vi "Updata LeafNumber.vi"(8 "error in (no error)":errorcluster caption="错误输入（无错误）", 11 "PanelLinkNode 输入":refnum<class "PanelLinkNode.lvclass"> caption="DNL_LabVIEW Object in") -> (0 "error out":errorcluster caption="错误输出", 2 "*Leafs":u8, 3 "PanelLinkNode 输出":refnum<class "PanelLinkNode.lvclass"> caption="DNL_LabVIEW Object out")   [LabVIEW 2013, in "PanelLinkNode.lvclass"]
uses:
  PanelLinkNode.lvclass
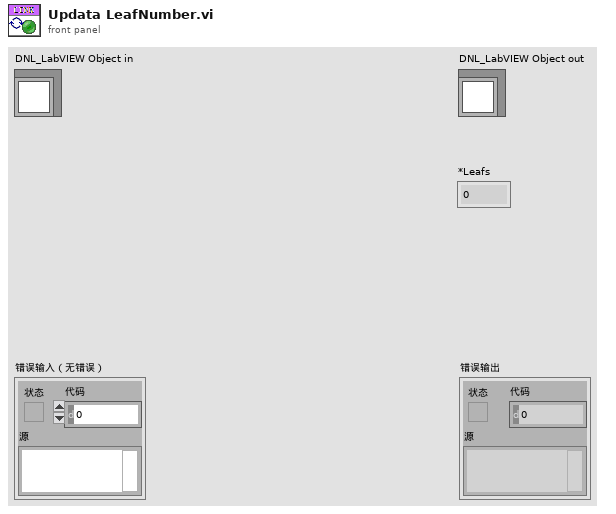
[diagram p1: front panel]
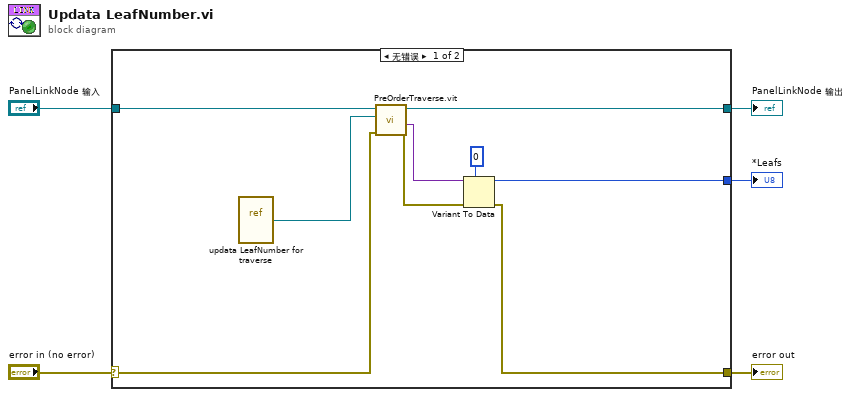
[diagram p0: block diagram]
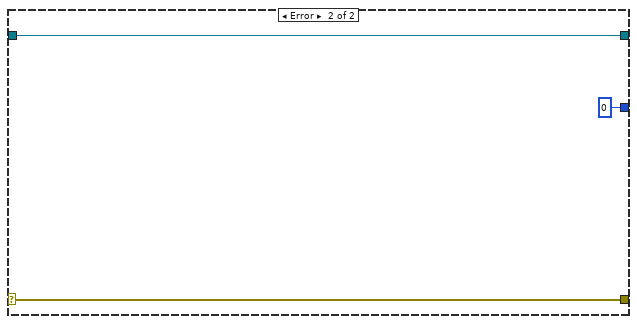
[diagram p2: hidden frame]
diagram:
  n1 = case shown="无错误" "error in (no error)" {
    selector: "error in (no error)" -> [w7 w17]
    tunnel: [w6 w17] -> w4
    tunnel: [w14 w16] -> w2
    tunnel: "PanelLinkNode 输入" -> [w9 w16]
    tunnel: [w11 u8 0] -> w1
    frame No Error {
      n2 = vi-ref "updata LeafNumber for traverse.vi"() -> (w10:refnum<vi>)
      n3 = call-dynamic "PreOrderTraverse.vit"("error in"=w7, "vi reference"=w10, "PanelLinkNode 输入"=w9) -> ("error out"=w8:errorcluster, "Data out"=w13:variant, "PanelLinkNode 输出"=w14:refnum<class "PanelLinkNode.lvclass">)  [unwired: 5 in, 1 out]
      n4 = Variant To Data(error in=w8, type=u8 0, Variant=w13) -> (data=w11:u8, error out=w6:errorcluster)
    }
    frame Error {
    }
  }
  "error out" <- w4
  "PanelLinkNode 输出" <- w2
  "*Leafs" <- w1
